vi "Pololu.Mgr - Save Config.vi"(8 "error in (no error)":errorcluster, 10 "Config Folder":path, 11 "PololuCtrl in":refnum<class "PololuCtrl.lvclass">) -> (0 "error out":errorcluster, 3 "PololuCtrl out":refnum<class "PololuCtrl.lvclass">)   [LabVIEW 2018, in "PololuCtrl.lvclass"]
uses:
  PololuCtrl.lvclass
  Utils/Errors/Error.Error Code List.ctl
  PololuCtrl.lvclass/PololuCtrl.ctl
  <vilib>/KATE/Files/File Utils.lvlib
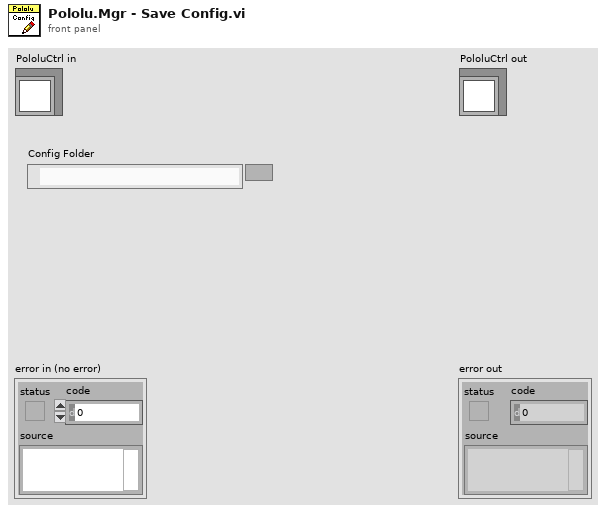
[diagram p1: front panel]
types:
  T1 = typedef "Error.Error Code List.ctl" = i32
  T2 = typedef "Pololu.Device Config.ctl" = cluster{"Chan":u8, "Accel":u16, "Speed":u16, "Positions":dbl[], "Range Info":T3}
  T3 = typedef "Pololu.Device Range Config.ctl" = cluster{"Min us":dbl, "Max us":dbl, "Min deg":dbl, "Max deg":dbl, "LStopDeg":dbl, "UStopDeg":dbl}
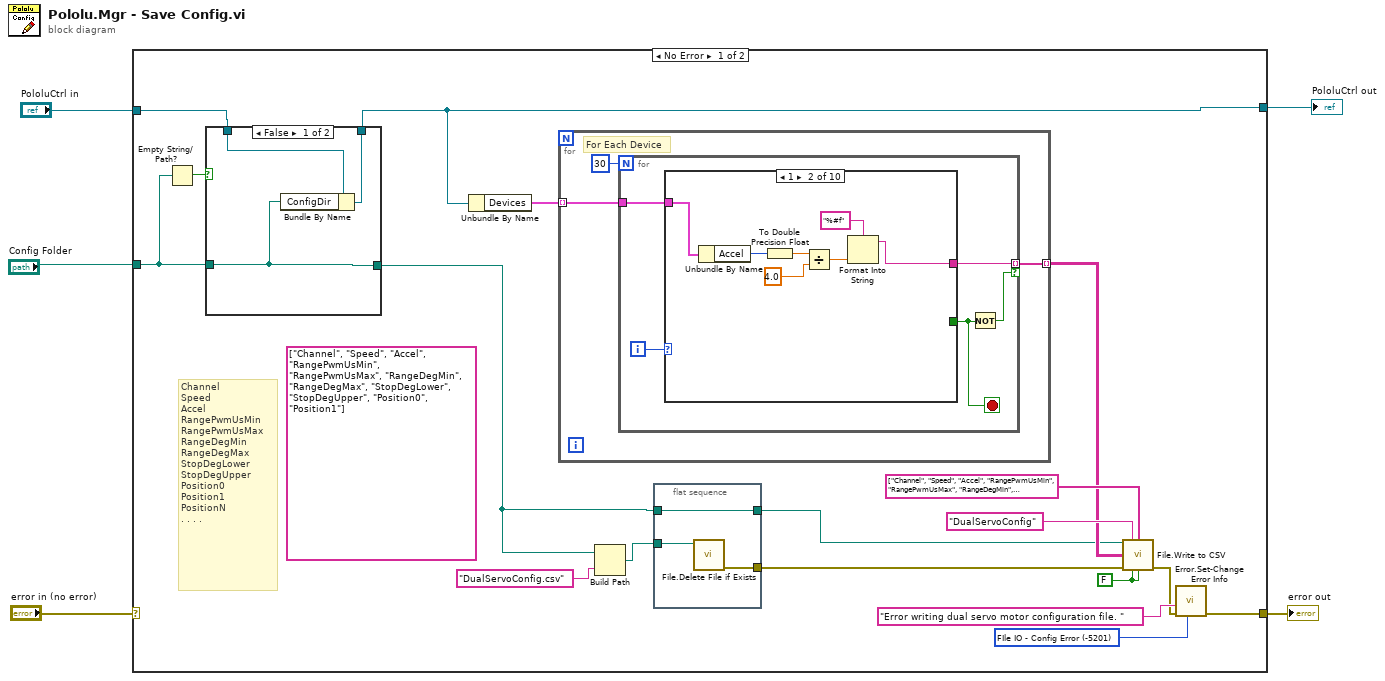
[diagram p0: block diagram]
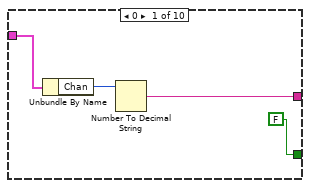
[diagram p2: hidden frame]
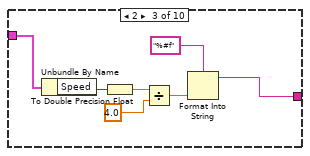
[diagram p3: hidden frame]
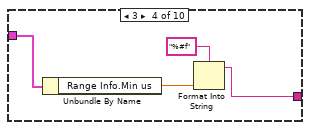
[diagram p4: hidden frame]
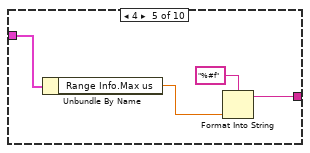
[diagram p5: hidden frame]
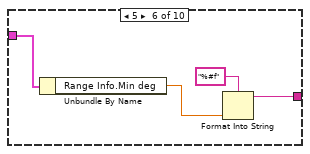
[diagram p6: hidden frame]
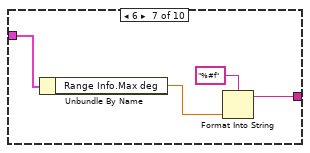
[diagram p7: hidden frame]
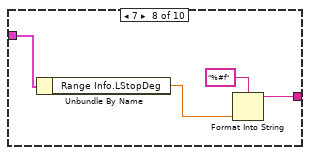
[diagram p8: hidden frame]
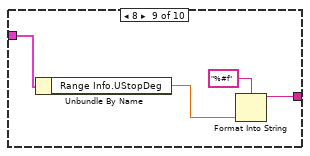
[diagram p9: hidden frame]
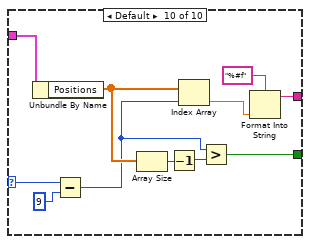
[diagram p10: hidden frame]
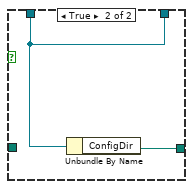
[diagram p11: hidden frame]
diagram:
  n1 = case shown="No Error" "error in (no error)" {
    selector: "error in (no error)" -> [_ w94]
    tunnel: [w23 w94] -> w4
    tunnel: [w16 w93] -> w2
    tunnel: "PololuCtrl in" -> [w19 w93]
    tunnel: "Config Folder" -> [w18 _]
    frame No Error {
      w12 = FALSE ("Append Time to Filename")
      (unwired) string[] ["Channel", "Speed", "Accel", "RangePwmUsMin", "RangePwmUsMax", "RangeDegMin", "RangeDegMax", "StopDegLower", "StopDegUpper", "Position0", "Position1"]
      w22 = T1 -5201 items=["No Error"=0, "Abort"=-2, "Misc"=-5000, "Fixture Error"=-5100, "File IO - General"=-5200, "FIle IO - Config Error"=-5201, "Instrument - General"=-5300, "Instrument - Serial Com"=-5301, "Instrument - Camera"=-5302, "Instrument - PS"=-5303, "Instrument - Oscilloscope"=-5304, "Instrument - Function Gen"=-5305, "Instrument - Load"=-5306, "Instrument - Meter"=-5307, "Instrument - Power Control"=-5308, "Instrument - Motion"=-5309, "Instrument - RF"=-5310, "System Exe"=-5400, "Image Processing"=-5500, "Communication"=-5600, "Script - Syntax Error"=-6000, "Script - Invalid Name or Param"=-6100, "Script - Timeout"=-6200, "Invalid Data"=-6300, "FW Update Error"=-6500] ("Std Code")
      # "Channel\nSpeed\nAccel\nRangePwmUsMin\nRangePwmUsMax\nRangeDegMin\nRangeDegMax\nStopDegLower\nStopDegUpper\nPosition0\nPosition1\nPositionN\n. . . ."
      n2 = Empty String/Path?(string/path=w18) -> (empty?=w20:bool)
      n3 = case shown="False" w20 {
        tunnel: [w90 w91] -> w16
        tunnel: w18 -> [w89 _]
        tunnel: w19 -> [w88 w91]
        tunnel: [w89 w92] -> w7
        frame False {
          n4 = Bundle By Name(cluster=w88, "ConfigDir"=w89) -> (w90:refnum<class "PololuCtrl.lvclass">)
        }
        frame True {
          n5 = Unbundle By Name(w91) -> ("ConfigDir"=w92:path)
        }
      }
      n6 = Unbundle By Name(w16) -> ("Devices"=w17:T2[])
      n7 = for {
        tunnel: w17 -> [w29] mode=indexing
        tunnel: [w28] -> w13 mode=indexing
        # "For Each Device"
        n8 = for {
          N: 30 -> [_]
          tunnel: w29 -> [w33]
          tunnel: [w32] -> w28 mode=indexing if=w31
          i -> [w34]
          stop <- w30 stop-if-true
          n9 = case shown="1" w34 {
            selector: w34 -> [_ _ _ _ _ _ _ _ _ w85]
            tunnel: w33 -> [w38 w45 w52 w56 w60 w64 w68 w72 w76 w87]
            tunnel: [w36 w39 w46 w53 w58 w62 w66 w70 w74 w78] -> w32
            tunnel: [FALSE _ _ _ _ _ _ _ _ w82] -> w30
            frame 0 {
              n10 = Unbundle By Name(w38) -> ("Chan"=w37:u8)
              n11 = Number To Decimal String(number=w37) -> (decimal integer string=w36:string)  [unwired: 1 in]
            }
            frame 1 {
              n12 = Unbundle By Name(w45) -> ("Accel"=w44:u16)
              n13 = To Double Precision Float(number=w44) -> (double precision float=w43:dbl)
              n14 = Divide(x=w43, y=4.0) -> (x/y=w41:dbl)
              n15 = Format Into String(format string="%#f", w41) -> (resulting string=w39:string)  [unwired: 2 in, 1 out]
            }
            frame 2 {
              n16 = Unbundle By Name(w52) -> ("Speed"=w47:u16)
              n17 = To Double Precision Float(number=w47) -> (double precision float=w51:dbl)
              n18 = Divide(x=w51, y=4.0) -> (x/y=w49:dbl)
              n19 = Format Into String(format string="%#f", w49) -> (resulting string=w46:string)  [unwired: 2 in, 1 out]
            }
            frame 3 {
              n20 = Unbundle By Name(w56) -> ("Range Info.Min us"=w54:dbl)
              n21 = Format Into String(format string="%#f", w54) -> (resulting string=w53:string)  [unwired: 2 in, 1 out]
            }
            frame 4 {
              n22 = Unbundle By Name(w60) -> ("Range Info.Max us"=w57:dbl)
              n23 = Format Into String(format string="%#f", w57) -> (resulting string=w58:string)  [unwired: 2 in, 1 out]
            }
            frame 5 {
              n24 = Unbundle By Name(w64) -> ("Range Info.Min deg"=w61:dbl)
              n25 = Format Into String(format string="%#f", w61) -> (resulting string=w62:string)  [unwired: 2 in, 1 out]
            }
            frame 6 {
              n26 = Unbundle By Name(w68) -> ("Range Info.Max deg"=w65:dbl)
              n27 = Format Into String(format string="%#f", w65) -> (resulting string=w66:string)  [unwired: 2 in, 1 out]
            }
            frame 7 {
              n28 = Unbundle By Name(w72) -> ("Range Info.LStopDeg"=w69:dbl)
              n29 = Format Into String(format string="%#f", w69) -> (resulting string=w70:string)  [unwired: 2 in, 1 out]
            }
            frame 8 {
              n30 = Unbundle By Name(w76) -> ("Range Info.UStopDeg"=w73:dbl)
              n31 = Format Into String(format string="%#f", w73) -> (resulting string=w74:string)  [unwired: 2 in, 1 out]
            }
            frame Default {
              n32 = Unbundle By Name(w87) -> ("Positions"=w86:dbl[])
              n33 = Subtract(x=w85, y=9) -> (x-y=w80:i32)
              n34 = Array Size(array=w86) -> (size(s)=w83:i32)
              n35 = Decrement(x=w83) -> (x-1=w81:i32)
              n36 = Index Array(array=w86, index=w80) -> (element=w77:dbl)
              n37 = Greater?(x=w80, y=w81) -> (0:w82:bool)
              n38 = Format Into String(format string="%#f", w77) -> (resulting string=w78:string)  [unwired: 2 in, 1 out]
            }
          }
          n39 = Not(x=w30) -> (.not. x?=w31:bool)
        }
      }
      n40 = Build Path(base path=w7, name or relative path="DualServoConfig.csv") -> (appended path=w8:path)
      n41 = flat-sequence {
        tunnel: [w26] -> w10
        tunnel: w8 -> [w25]
        tunnel: w7 -> [w24]
        tunnel: [w24] -> w6
        frame #0 {
          n42 = call "File.Delete File if Exists.vi"("Path"=w25) -> ("error out"=w26:errorcluster)  [unwired: 9 in, 1 out]
        }
      }
      n43 = call <vilib>:"File.Write to CSV.vi"("Folder"=w6, "FileRootName"="DualServoConfig", "Header"=string[] ["Channel", "Speed", "Accel", "RangePwmUsMin", "RangePwmUsMax", "RangeDegMin", "RangeDegMax", "StopDegLower", "StopDegUpper", "Position0", "Position1"], "2D"=w13, "error in"=w10, "Append Time to Filename"=w12, "Append Date to Filename"=w12) -> ("error out"=w11:errorcluster)  [unwired: 7 in, 1 out]
      n44 = call "Error.Set-Change Error Info.vi"("Std Code"=w22, "error in"=w11, "Description"="Error writing dual servo motor configuration file. ") -> ("error out"=w23:errorcluster)  [unwired: 8 in]
    }
    frame Error {
    }
  }
  "error out" <- w4
  "PololuCtrl out" <- w2
